vi "Close.vi"(8 "error in (no error)":errorcluster, 11 "SpecA_ESA in":refnum<class "SpecA_ESA.lvclass">) -> (0 "error out":errorcluster)   [LabVIEW 2014, in "SpecA_ESA.lvclass"]
uses:
  SpecA_ESA.lvclass
  SpecA_ESA.lvclass/SpecA_ESA.ctl
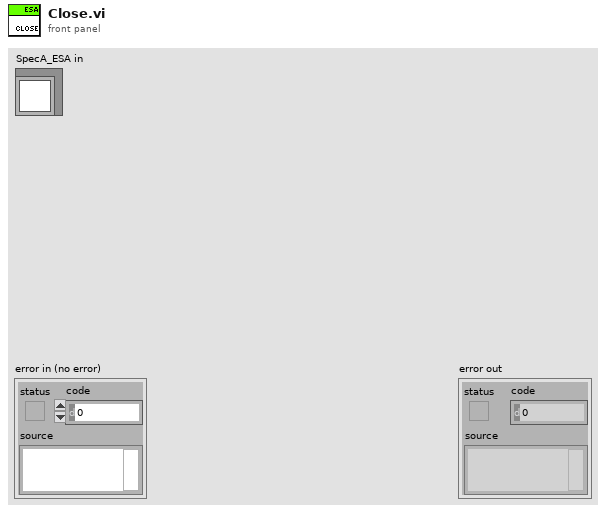
[diagram p1: front panel]
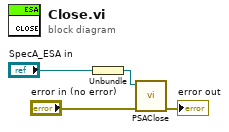
[diagram p0: block diagram]
diagram:
  n1 = Unbundle("SpecA_ESA in") -> (w2:refnum<visa-resource-name>)
  n2 = call "PSAClose.vi"("error in (no error)"="error in (no error)", "PSA In"=w2) -> ("error out"=→"error out":errorcluster)  [unwired: 9 in]
